vi "API get solen statue.vi"(11 "solenstatue input":i32[](array[numeric])) -> (3 "solenstatue output":i32[](array[numeric]))   [LabVIEW 2011, in "API DYM.lvlib"]
uses:
  API DYM.lvlib
  DyMechnicalPlatform.dll
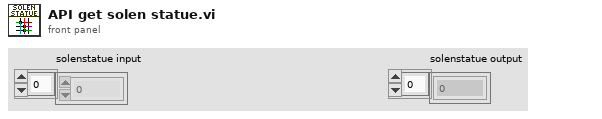
[diagram p1: front panel]
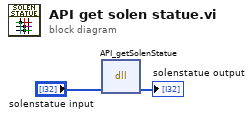
[diagram p0: block diagram]
diagram:
  n1 = dll-call lib="PTH1Xabs D可重构机电平台项目DemoLabViewDYSYSAPIDyMechnicalPlatform.dll" fn="API_getSolenStatue"("solenstatue"="solenstatue input") -> ("solenstatue"=→"solenstatue output":i32[])  [unwired: 4 in, 2 out]
